vi "GT_SetStopIo.vi"(6 "inputTypeIndex":i16, 8 "inputType":i16(ring) items=["Limit_Positive", "Limit_Negative", "Alarm", "Home", "Gpi", "Arrive"], 9 "stopType":i16(ring) items=["Abrupt", "Smooth"], 10 "axis in":i16, 11 "rtn_In":cluster{"rtn":i16, "Func":string}) -> (2 "axis out":i16, 3 "rtn_Out":cluster{"rtn":i16, "Func":string})   [LabVIEW 2014]
uses:
  VC6/gts.dll
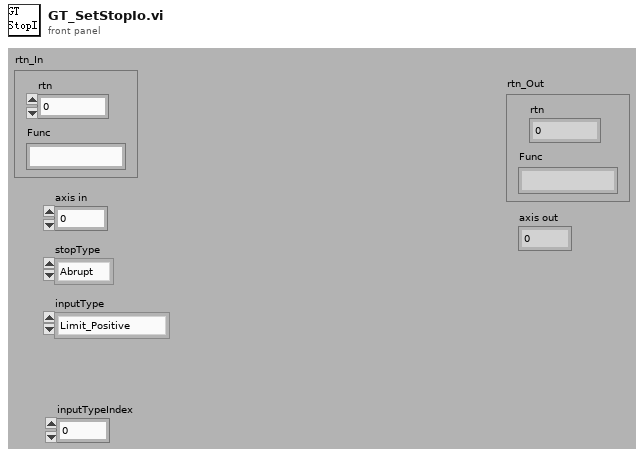
[diagram p1: front panel]
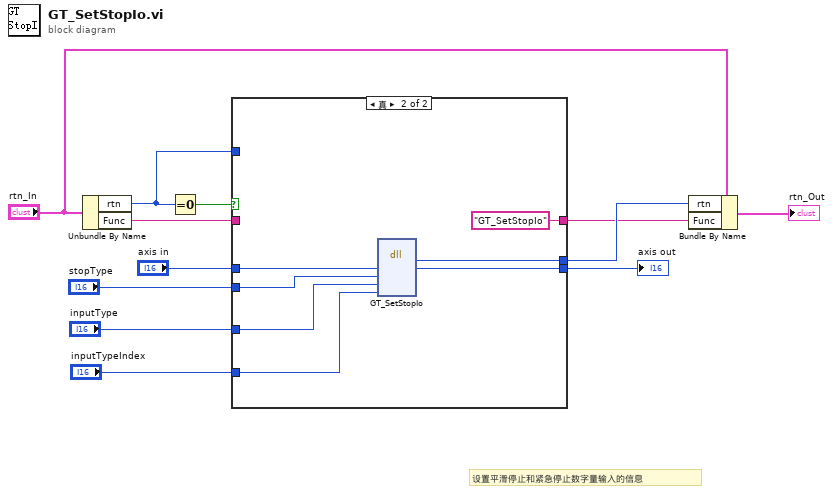
[diagram p0: block diagram]
diagram:
  # "设置平滑停止和紧急停止数字量输入的信息"
  n1 = Unbundle By Name("rtn_In") -> ("rtn"=w6:i16, "Func"=w8:string)
  n2 = Equal To 0?(x=w6) -> (x = 0?=w12:bool)
  n3 = case shown="真" w12 {
    tunnel: [w14 w22] -> w9
    tunnel: w8 -> [w15 _]
    tunnel: [w15 "GT_SetStopIo" ("Func")] -> w7
    tunnel: w6 -> [w14 _]
    tunnel: "axis in" -> [w13 w20]
    tunnel: "stopType" -> [_ w19]
    tunnel: "inputType" -> [_ w18]
    tunnel: "inputTypeIndex" -> [_ w17]
    tunnel: [w13 w16] -> w1
    frame False {
    }
    frame True {
      n4 = dll-call lib="PTH2Fabs DNewGTS AC-800LWin7版源程序-20170926gts85VC6gts.dll" fn="GT_SetStopIo"("axis"=w20, "stopType"=w19, "inputType"=w18, "inputTypeIndex"=w17) -> ("rtn"=w22:i16, "axis"=w16:i16)  [unwired: 6 in, 2 out]
    }
  }
  "axis out" <- w1
  n5 = Bundle By Name(cluster="rtn_In", "rtn"=w9, "Func"=w7) -> (→"rtn_Out":cluster{"rtn":i16, "Func":string})
